vi "Send Message to caller.vi"(8 "error in (no error)":errorcluster, 10 "Message Data":variant, 11 "Domino Laser module Class in":refnum<class "Domino Laser module Class.lvclass">) -> (0 "error out":errorcluster, 3 "Domino Laser module Class out":refnum<class "Domino Laser module Class.lvclass">)   [LabVIEW 2015, in "Domino LM.lvlib" / "Domino Laser module Class.lvclass"]
uses:
  CTRLS/Domino Laser module Class.lvclass
  ARCH/Message Queue/Message Cluster.ctl
  CTRLS/Domino Laser module Class.lvclass/Domino Laser module Class.ctl
  ARCH/Message Queue/Message Queue.lvlib
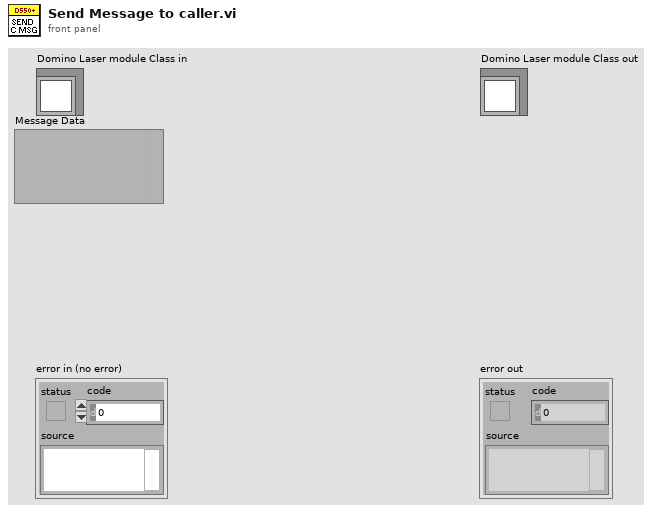
[diagram p1: front panel]
types:
  T1 = typedef "Message Queue.lvlib/Message Cluster.ctl" = cluster{"Message":string, "Message Data":variant}
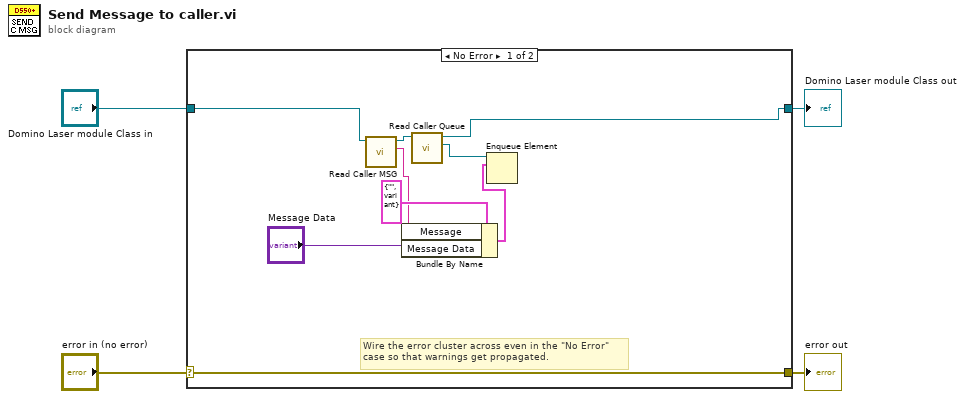
[diagram p0: block diagram]
diagram:
  n1 = case shown="No Error" "error in (no error)" {
    selector: "error in (no error)" -> [w13 w15]
    tunnel: [w13 w15] -> w3
    tunnel: [w6 w14] -> w1
    tunnel: "Domino Laser module Class in" -> [w10 w14]
    frame No Error {
      # "Wire the error cluster across even in the \"No Error\"\ncase so that warnings get propagated."
      n2 = call "Read Caller MSG.vi"("Domino Laser module Class in"=w10) -> ("Caller MSG"=w8:string, "Domino Laser module Class out"=w11:refnum<class "Domino Laser module Class.lvclass">)  [unwired: 8 in, 1 out]
      n3 = Bundle By Name(cluster=T1 {"Message"="", "Message Data"=variant} ("element"), "Message"=w8, "Message Data"="Message Data") -> (w5:T1)
      n4 = call "Read Caller Queue.vi"("Domino Laser module Class in"=w11) -> ("Caller Queue"=w12:refnum<queue>, "Domino Laser module Class out"=w6:refnum<class "Domino Laser module Class.lvclass">)  [unwired: 8 in, 1 out]
      n5 = Enqueue Element(queue=w12, element=w5) -> ()  [unwired: 2 in, 3 out]
    }
    frame Error {
    }
  }
  "error out" <- w3
  "Domino Laser module Class out" <- w1
